vi "Step1.vi"(1 "군집_데이터":i32[](array[numeric]), 2 "클러스터":i32) -> (0 "ALL_U":ext[][](array[numeric]))   [LabVIEW 2011]
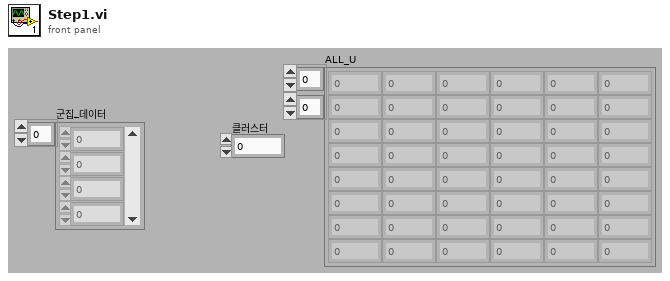
[diagram p1: front panel]
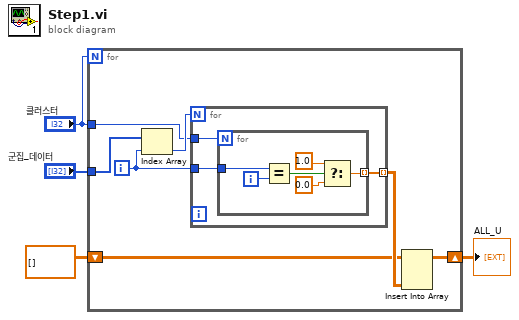
[diagram p0: block diagram]
diagram:
  n1 = for {
    N: "클러스터" -> [_]
    tunnel: "군집_데이터" -> [w11]
    tunnel: "클러스터" -> [w8]
    shift-right: [w5] -> w1
    shift-left: dbl[][] [] -> [w6]
    i -> [w9]
    n2 = Index Array(array=w11, index=w9) -> (element=w10:i32)
    n3 = for {
      N: w10 -> [_]
      tunnel: w9 -> [w13]
      tunnel: w8 -> [w14]
      tunnel: [w12] -> w7 mode=indexing
      n4 = for {
        N: w14 -> [_]
        tunnel: w13 -> [w19]
        tunnel: [w15] -> w12 mode=indexing
        i -> [w20]
        n5 = Equal?(x=w19, y=w20) -> (x = y?=w18:bool)
        n6 = Select(t=1.0, s=w18, f=0.0) -> (s? t:f=w15:dbl)
      }
    }
    n7 = Insert Into Array(array=w6, new element=w7) -> (w5:dbl[][])  [unwired: 2 in]
  }
  "ALL_U" <- w1
